vi "haha.vi"() -> ()   [LabVIEW 2021]
uses:
  <vilib>/express/express analysis/Spectral/Block/exnSpectralBlock spectral measurements PSD poly.vi
  <vilib>/express/express analysis/Spectral/Block/exnSpectralBlock spectral measurements PSD DDT.vi
  <vilib>/express/express analysis/Spectral/XNode/ExpressSpectralMeasurementsBlockNode.xnode
panel:
  in  "rate":dbl=1000.0
  in  "number of samples":i32=100
  in  "device name":tag="Dev1"
  out "Waveform Graph":dynamicdata(graph)
  out "data":dynamicdata(graph)
  in  "stop":bool
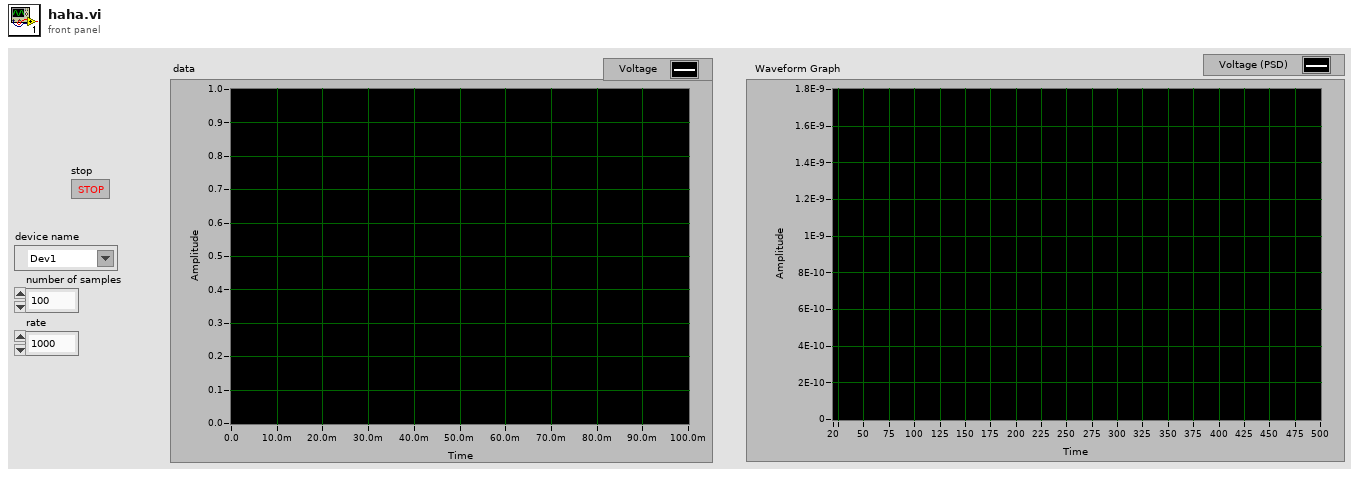
[diagram p1: front panel]
types:
  T1 = cluster{"averaging mode":u16, "weighting mode":u16, "number of averages":u32}
  T2 = cluster{"dB On (F)":bool, "unwrap phase (F)":bool, "convert to degree (F)":bool}
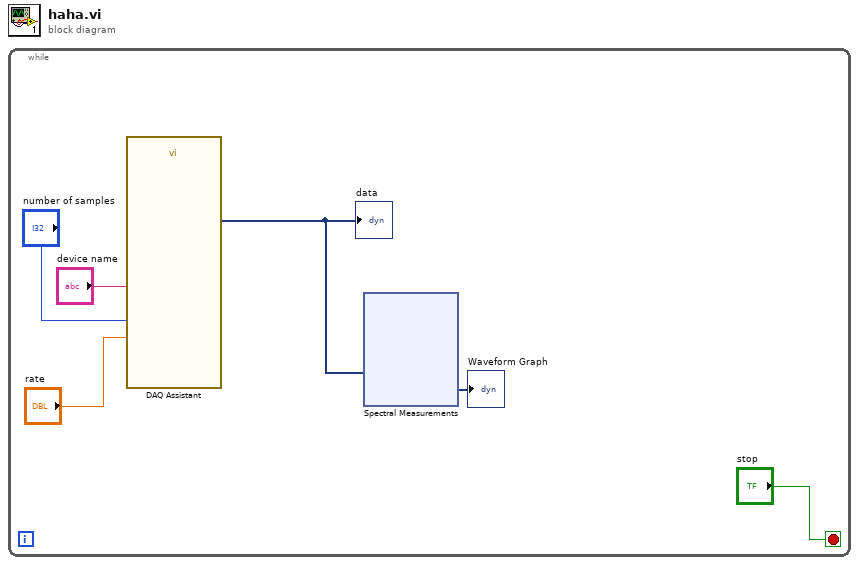
[diagram p0: block diagram]
diagram:
  n1 = while {
    stop <- "stop" stop-if-true
    n2 = call "DAQ Assistant"("rate"="rate", "number of samples"="number of samples", "device name"="device name") -> ("data"=w4:dynamicdata)  [unwired: 13 in, 3 out]
    "data" <- w4
    n3 = xnode "Spectral Measurements"("Signals"=w4) -> ("PSD"=→"Waveform Graph":dynamicdata)  [unwired: 1 in, 1 out]
  }
